vi "Brain.vi"() -> ()   [LabVIEW 2017]
uses:
  <vilib>/OPCUA/controls/NodeId.ctl
  <vilib>/OPCUA/controls/Write Status.ctl
  <vilib>/Utility/file.llb/Read Delimited Spreadsheet (string).vi
  <vilib>/Utility/file.llb/Write Delimited Spreadsheet (string).vi
  <vilib>/OPCUA/client/Multiple Write Double Array.vi
  <vilib>/Utility/file.llb/Write Delimited Spreadsheet (DBL).vi
  <resource>/objmgr/ni.dex.rc
  <vilib>/OPCUA/NI OPC UA Client.lvlib
panel:
  in  "error in (no error)":errorcluster
  in  "VFD Stop":bool
  in  "Shutdown":bool
  out "Remote VI Error Messages":string
  in  "Node Status":u16
  in  "Time Stamp":timestamp
  out "Error Out":errorcluster
  in  "Stop DAQ":bool
  out "DAQ?":bool
  out "Available Elements for Reading":i32
  out "Number of Disconnections":u32
  out "System Loop Time (ms)":u32
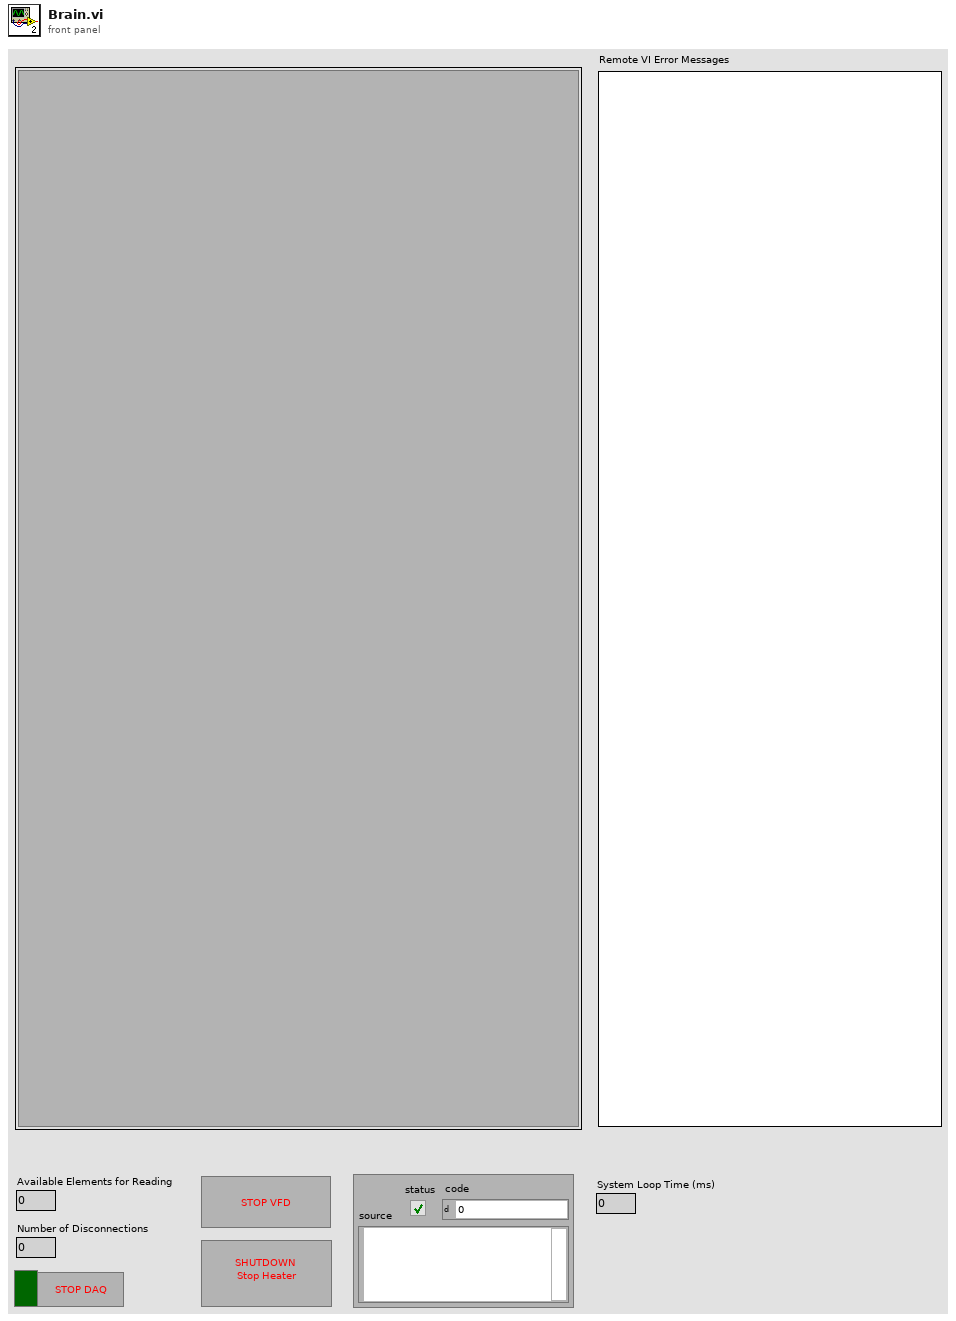
[diagram p1: front panel]
types:
  T1 = typedef "OPC UA Client Refnum.ctl" = refnum<k21>
  T2 = typedef "NodeId.ctl" = string
  T3 = typedef "Write Status.ctl" = u32
  T4 = cluster{"node ID":T2, "value":dbl[], "timestamp (current time)":timestamp, "node status":T3}
  T5 = cluster{"node ID":T2, "value":dbl[], "timestamp (current time)":timestamp, "node status":T3}[]
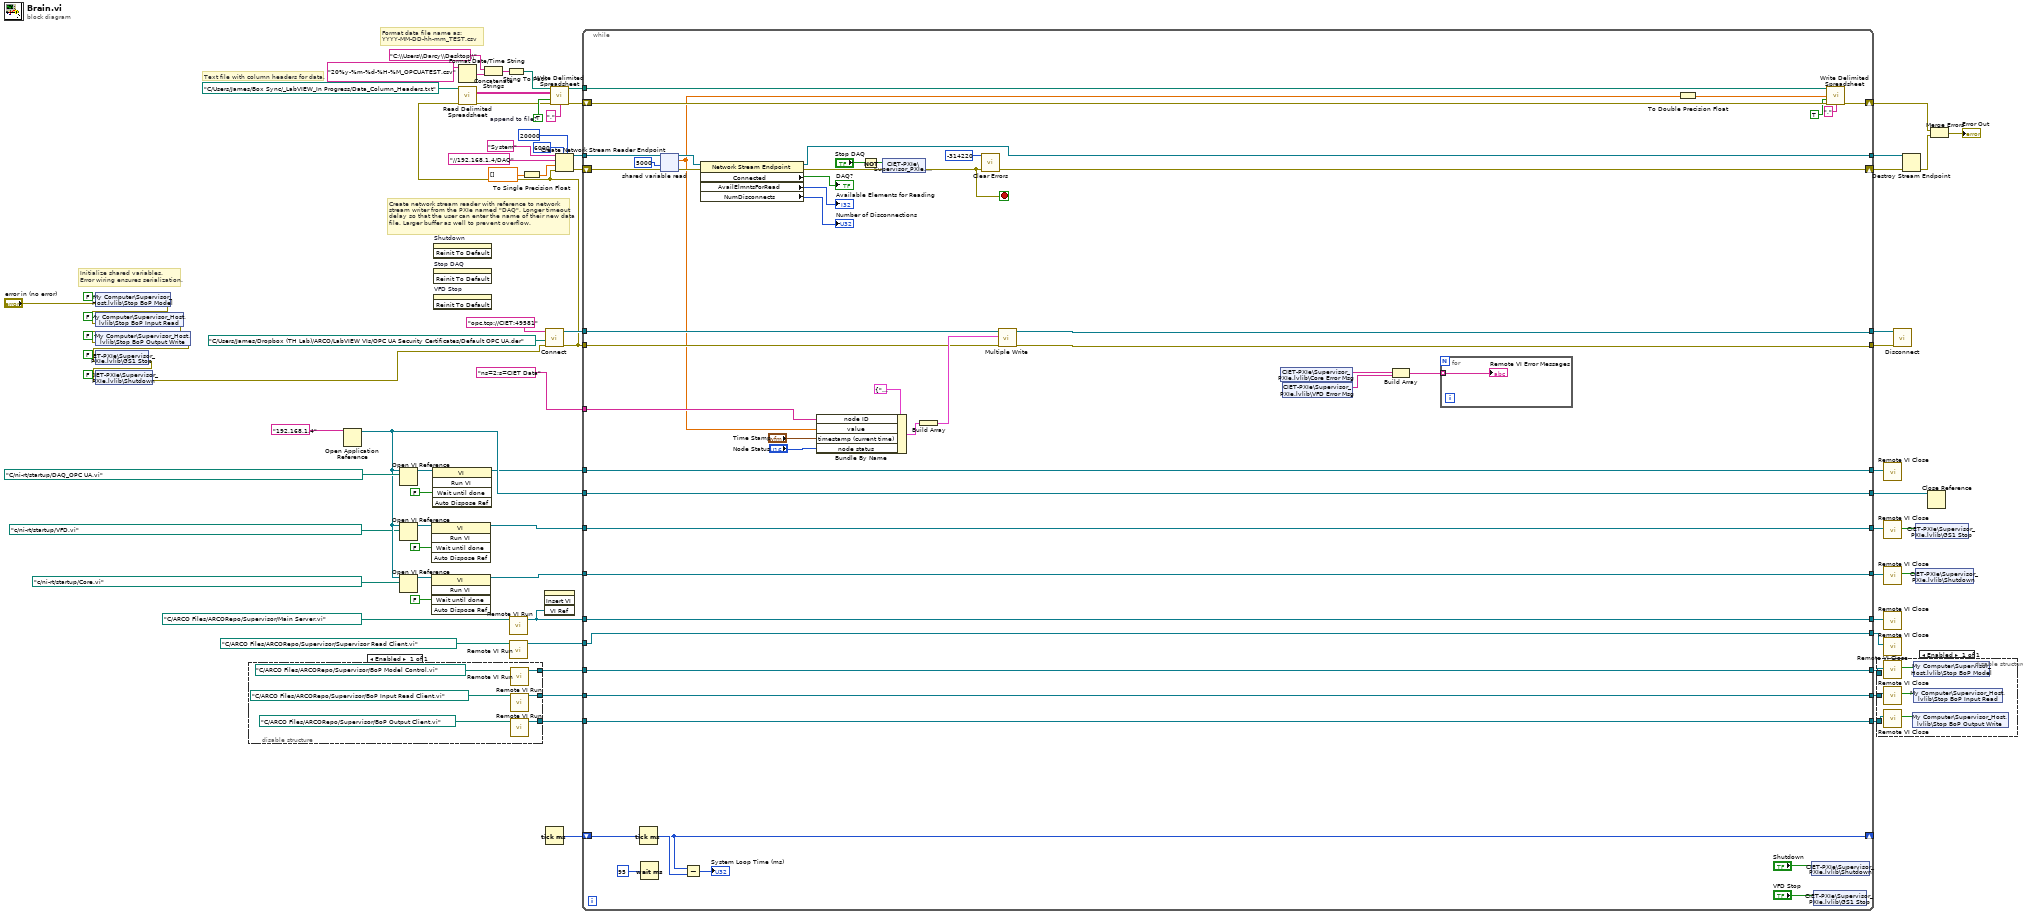
[diagram p0: block diagram]
diagram:
  w63 = TRUE  # append to file?
  # "Initialize shared variables.\nError wiring ensures serialization."
  # "Format data file name as:\nYYYY-MM-DD-hh-mm_TEST.csv"
  # "Create network stream reader with reference to network\nstream writer from the PXIe named \"DAQ\". Longer timeout\ndelay so that the user can enter the name of their new data\nfile. Larger buffer as well to prevent overflow."
  # "Text file with column headers for data."
  n1 = shared-variable "My Computer\\Supervisor_Host.lvlib\\Stop BoP Model"(FALSE ("Stop BoP Model"), error in="error in (no error)") -> (error out=w12:errorcluster)
  n2 = shared-variable "My Computer\\Supervisor_Host.lvlib\\Stop BoP Input Read"(FALSE ("Stop BoP Input Read"), error in=w12) -> (error out=w11:errorcluster)
  n3 = shared-variable "My Computer\\Supervisor_Host.lvlib\\Stop BoP Output Write"(FALSE ("Stop BoP Output Write"), error in=w11) -> (error out=w10:errorcluster)
  n4 = shared-variable "CIET-PXIe\\Supervisor_PXIe.lvlib\\GS1 Stop"(FALSE ("GS1 Stop"), error in=w10) -> (error out=w9:errorcluster)
  n5 = shared-variable "CIET-PXIe\\Supervisor_PXIe.lvlib\\Shutdown"(FALSE ("Shutdown"), error in=w9) -> (error out=w8:errorcluster)
  n6 = disable-structure shown="Enabled" {
    disable-tunnel: [w79] -> w19
    disable-tunnel: [w78] -> w17
    disable-tunnel: [w77] -> w15
    frame Enabled {
      n7 = call "Remote VI Run.vi"("VI Path"=path "C:/ARCO Files/ARCORepo/Supervisor/BoP Model Control.vi" ("vi path")) -> ("VI Reference"=w79:refnum<vi>)  [unwired: 10 in]
      n8 = call "Remote VI Run.vi"("VI Path"=path "C:/ARCO Files/ARCORepo/Supervisor/BoP Input Read Client.vi" ("vi path")) -> ("VI Reference"=w78:refnum<vi>)  [unwired: 10 in]
      n9 = call "Remote VI Run.vi"("VI Path"=path "C:/ARCO Files/ARCORepo/Supervisor/BoP Output Client.vi" ("vi path")) -> ("VI Reference"=w77:refnum<vi>)  [unwired: 10 in]
    }
  }
  n10 = Open Application Reference(11:"192.168.1.4" ("machine name (\"\":  open local reference)")) -> (3:w36:refnum<vi>)  [unwired: 3 in, 1 out]
  n11 = Open VI Reference(application reference (local)=w36, vi path=path "C:/ni-rt/startup/DAQ_OPC UA.vi") -> (vi reference=w33:refnum<vi>)  [unwired: 4 in, 1 out]
  n12 = Open VI Reference(application reference (local)=w36, vi path=path "c:/ni-rt/startup/VFD.vi") -> (vi reference=w31:refnum<vi>)  [unwired: 4 in, 1 out]
  n13 = Open VI Reference(application reference (local)=w36, vi path=path "c:/ni-rt/startup/Core.vi") -> (vi reference=w29:refnum<vi>)  [unwired: 4 in, 1 out]
  n14 = invoke class="VI" method="Run VI"(reference=w31, "Wait until done"=FALSE ("Wait Until Done")) -> (reference out=w30:refnum<vi>)  [unwired: 3 in, 4 out]
  n15 = invoke class="VI" method="Run VI"(reference=w29, "Wait until done"=FALSE ("Wait Until Done")) -> (reference out=w28:refnum<vi>)  [unwired: 3 in, 4 out]
  n16 = invoke class="VI" method="Run VI"(reference=w33, "Wait until done"=FALSE ("Wait Until Done")) -> (reference out=w32:refnum<vi>)  [unwired: 3 in, 4 out]
  n17 = invoke on="Shutdown" class="Bool (strict)" method="Reinit To Default"() -> ()  [unwired: 3 in, 3 out]
  n18 = invoke on="Stop DAQ" class="Bool (strict)" method="Reinit To Default"() -> ()  [unwired: 3 in, 3 out]
  n19 = invoke on="VFD Stop" class="Bool (strict)" method="Reinit To Default"() -> ()  [unwired: 3 in, 3 out]
  n20 = Format Date/Time String(time format string (%c)="20%y-%m-%d-%H-%M_OPCUATEST.csv") -> (date/time string=w53:string)  [unwired: 2 in]
  n21 = Concatenate Strings("C:\\Users\\Darcy\\Desktop\\" ("string"), w53) -> (w55:string)
  n22 = String To Path(string=w55) -> (path=w52:path)
  n23 = call "Remote VI Run.vi"("VI Path"=path "C:/ARCO Files/ARCORepo/Supervisor/Main Server.vi" ("vi path")) -> ("VI Reference"=w38:refnum<vi>)  [unwired: 10 in]
  n24 = call "Remote VI Run.vi"("VI Path"=path "C:/ARCO Files/ARCORepo/Supervisor/Supervisor Read Client.vi" ("vi path")) -> ("VI Reference"=w21:refnum<vi>)  [unwired: 10 in]
  n25 = To Single Precision Float(number=dbl[] []) -> (single precision float=w74:sgl[])
  n26 = invoke on="Sub Panel" class="SubPnl" method="Insert VI"("VI Ref"=w38) -> ()  [unwired: 3 in, 4 out]
  n27 = call <vilib>:"Connect.vi"("error in (no error)"=w8, "client certificate file"=path "C:/Users/James/Dropbox (TH Lab)/ARCO/LabVIEW VIs/OPC UA Security Certificates/Default OPC UA.der", "server endpoint URL"="opc.tcp://CIET:49581") -> ("error out"=w1:errorcluster, "OPC UA client refnum out"=w48:T1)  [unwired: 6 in, 1 out]
  n28 = call-poly <vilib>:"Read Delimited Spreadsheet.vi"("file path (dialog if empty)"=path "C:/Users/James/Box Sync/_LabVIEW_In Progress/Data_Column_Headers.txt", "error in (no error)"=w1) -> ("all rows"=w66:string[][], "error out"=w61:errorcluster)  [unwired: 8 in, 4 out]
  n29 = Tick Count (ms)() -> (millisecond timer value=w51:u32)
  n30 = call-poly <vilib>:"Write Delimited Spreadsheet.vi"("file path (dialog if empty)"=w52, "2D data"=w66, "append to file? (new file:F)"=w63, "error in (no error)"=w61, "delimiter (\\t)"=",") -> ("new file path (Not A Path if cancelled)"=w62:path, "error out"=w60:errorcluster)  [unwired: 9 in]
  n31 = Create Network Stream Reader Endpoint(5:20000 ("timeout in ms (-1)"), 7:6000 ("reader buffer size"), 8:w1, 9:w74, 10:"//192.168.1.4/DAQ" ("writer url"), 11:"System" ("reader name")) -> (0:w71:errorcluster, 3:w70:refnum<k21>)  [unwired: 1 in]
  n32 = while {
    shift-right: [w121] -> w69
    shift-left: w71 -> [w129]
    tunnel: w70 -> [w130]
    tunnel: [w120] -> w68
    tunnel: w62 -> [w116]
    shift-right: [w114] -> w59
    shift-left: w60 -> [w115]
    shift-right: [w109] -> _
    shift-left: w51 -> [w110]
    tunnel: w48 -> [w104]
    tunnel: w1 -> [w103]
    tunnel: "ns=2;s=CIET Data" -> [w102]
    tunnel: [w85] -> w46
    tunnel: [w84] -> w45
    tunnel: w32 -> [w101]
    tunnel: [w101] -> w43
    tunnel: w36 -> [w100]
    tunnel: [w100] -> w42
    tunnel: w30 -> [w99]
    tunnel: [w99] -> w41
    tunnel: w28 -> [w98]
    tunnel: [w98] -> w40
    tunnel: w38 -> [w97]
    tunnel: [w97] -> w39
    tunnel: w21 -> [w89]
    tunnel: [w89] -> w20
    tunnel: w19 -> [w88]
    tunnel: [w88] -> w18
    tunnel: w17 -> [w87]
    tunnel: [w87] -> w16
    tunnel: w15 -> [w86]
    tunnel: [w86] -> w14
    stop <- w119 stop-if-true
    n33 = Tick Count (ms)() -> (millisecond timer value=w109:u32)
    n34 = Wait (ms)(milliseconds to wait=u32 95) -> ()  [unwired: 1 out]
    n35 = shared-variable-read(w130, w129, 5000 ("timeout ms (-1)")) -> (w126:refnum<k21>, w124:errorcluster, w83:sgl[])  [unwired: 1 out]
    n36 = Subtract(x=w109, y=w110) -> (x-y=→"System Loop Time (ms)":u32)
    n37 = property class="Network Stream Endpoint"(reference=w126, error in=w124) -> (reference out=w120:refnum<k21>, error out=w125:errorcluster, "Connected"=→"DAQ?":bool, "AvailElmntsForRead"=→"Available Elements for Reading":i32, "NumDisconnects"=→"Number of Disconnections":u32)
    n38 = Bundle By Name(cluster=T4 {"node ID"="", "value"=[], "timestamp (current time)"=timestamp(0 s since 1904-01-01), "node status"=0} ("request"), "node ID"=w102, "value"=w83, "timestamp (current time)"="Time Stamp", "node status"="Node Status") -> (w106:T4)
    n39 = Not(x="Stop DAQ") -> (.not. x?=w128:bool)
    n40 = shared-variable "CIET-PXIe\\Supervisor_PXIe.lvlib\\DAQ?"(w128, error in=w125) -> (error out=w119:errorcluster)
    n41 = Build Array(w106) -> (w105:T5)
    n42 = call <vilib>:"Clear Errors.vi"("error in (no error)"=w119, "specific error code to clear (0: all)"=-314220) -> ("error out"=w121:errorcluster)  [unwired: 4 in, 1 out]
    n43 = call-poly <vilib>:"Multiple Write.vi"("error in (no error)"=w103, "requests"=w105, "OPC UA client refnum in"=w104) -> ("error out"=w84:errorcluster, "OPC UA client refnum out"=w85:T1)  [unwired: 5 in, 2 out]
    n44 = shared-variable "CIET-PXIe\\Supervisor_PXIe.lvlib\\Core Error Msg"() -> (w96:string)  [unwired: 1 in, 1 out]
    n45 = shared-variable "CIET-PXIe\\Supervisor_PXIe.lvlib\\VFD Error Msg"() -> (w95:string)  [unwired: 1 in, 1 out]
    n46 = Build Array(w96, w95) -> (w94:string[])
    n47 = for {
      tunnel: w94 -> [w133] mode=indexing
      "Remote VI Error Messages" <- w133
    }
    n48 = To Double Precision Float(number=w83) -> (double precision float=w111:dbl[])
    n49 = shared-variable "CIET-PXIe\\Supervisor_PXIe.lvlib\\Shutdown"("Shutdown") -> ()  [unwired: 1 in, 1 out]
    n50 = shared-variable "CIET-PXIe\\Supervisor_PXIe.lvlib\\GS1 Stop"("VFD Stop") -> ()  [unwired: 1 in, 1 out]
    n51 = call-poly <vilib>:"Write Delimited Spreadsheet.vi"("file path (dialog if empty)"=w116, "1D data"=w111, "append to file? (new file:F)"=TRUE, "error in (no error)"=w115, "delimiter (\\t)"="," ("delimiter (\\t)")) -> ("error out"=w114:errorcluster)  [unwired: 9 in, 1 out]
  }
  n52 = disable-structure shown="Enabled" {
    disable-tunnel: w18 -> [w139]
    disable-tunnel: w16 -> [w138]
    disable-tunnel: w14 -> [w137]
    frame Enabled {
      n53 = call "Remote VI Close.vi"("reference"=w139) -> ("SubVI Stop"=w135:bool)  [unwired: 10 in]
      n54 = call "Remote VI Close.vi"("reference"=w138) -> ("SubVI Stop"=w134:bool)  [unwired: 10 in]
      n55 = call "Remote VI Close.vi"("reference"=w137) -> ("SubVI Stop"=w136:bool)  [unwired: 10 in]
      n56 = shared-variable "My Computer\\Supervisor_Host.lvlib\\Stop BoP Output Write"(w136) -> ()  [unwired: 1 in, 1 out]
      n57 = shared-variable "My Computer\\Supervisor_Host.lvlib\\Stop BoP Model"(w135) -> ()  [unwired: 1 in, 1 out]
      n58 = shared-variable "My Computer\\Supervisor_Host.lvlib\\Stop BoP Input Read"(w134) -> ()  [unwired: 1 in, 1 out]
    }
  }
  n59 = call "Remote VI Close.vi"("reference"=w43) -> ()  [unwired: 10 in, 1 out]
  n60 = call "Remote VI Close.vi"("reference"=w41) -> ("SubVI Stop"=w13:bool)  [unwired: 10 in]
  n61 = call "Remote VI Close.vi"("reference"=w40) -> ("SubVI Stop"=w24:bool)  [unwired: 10 in]
  n62 = call "Remote VI Close.vi"("reference"=w39) -> ()  [unwired: 10 in, 1 out]
  n63 = call "Remote VI Close.vi"("reference"=w20) -> ()  [unwired: 10 in, 1 out]
  n64 = call <vilib>:"Disconnect.vi"("error in (no error)"=w45, "OPC UA client refnum in"=w46) -> ()  [unwired: 9 in, 1 out]
  n65 = Destroy Stream Endpoint(8:w69, 11:w68) -> (0:w58:errorcluster)
  n66 = shared-variable "CIET-PXIe\\Supervisor_PXIe.lvlib\\GS1 Stop"(w13) -> ()  [unwired: 1 in, 1 out]
  n67 = shared-variable "CIET-PXIe\\Supervisor_PXIe.lvlib\\Shutdown"(w24) -> ()  [unwired: 1 in, 1 out]
  n68 = Close Reference(reference=w42) -> ()  [unwired: 1 in, 1 out]
  n69 = Merge Errors(w59, w58) -> (→"Error Out":errorcluster)
